vi "Set Cell_row_string.vi"(7 "Value":string, 8 "error in (no error)":errorcluster, 9 "Column":i32, 11 "Row":refnum<k24>) -> (0 "error out":errorcluster, 3 "Row Out":refnum<k24>)   [LabVIEW 2013]
uses:
  C:/PhaeronGit/LVNPOI/Resources/NPOI 2.1.1 dotnet2/NPOI.dll
  Resources/NPOI 2.1.1 dotnet2/NPOI.dll
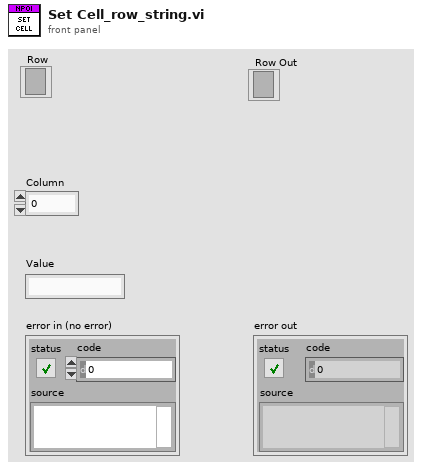
[diagram p1: front panel]
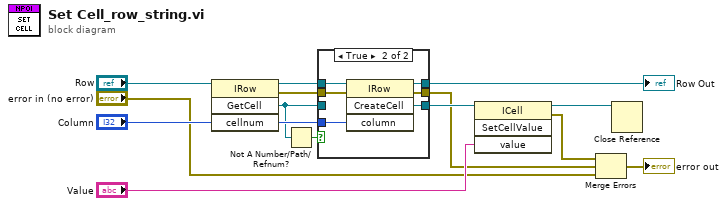
[diagram p0: block diagram]
diagram:
  n1 = invoke class="IRow" method="GetCell"(reference="Row", "cellnum"="Column") -> (reference out=w8:refnum<k24>, error out=w7:errorcluster, "GetCell"=w4:refnum<k24>)  [unwired: 2 in, 1 out]
  n2 = Not A Number/Path/Refnum?(number/path/refnum=w4) -> (NaN/Path/Refnum?=w5:bool)
  n3 = case shown="True" w5 {
    tunnel: w4 -> [w16 _]
    tunnel: [w16 w22] -> w9
    tunnel: "Column" -> [_ w21]
    tunnel: w8 -> [w15 w20]
    tunnel: [w15 w19] -> w1
    tunnel: [_ w18] -> w6
    tunnel: w7 -> [_ w17]
    frame False {
    }
    frame True {
      n4 = invoke class="IRow" method="CreateCell"(reference=w20, error in=w17, "column"=w21) -> (reference out=w19:refnum<k24>, error out=w18:errorcluster, "CreateCell"=w22:refnum<k24>)  [unwired: 1 in, 1 out]
    }
  }
  "Row Out" <- w1
  n5 = invoke class="ICell" method="SetCellValue"(reference=w9, "value"="Value") -> (reference out=w13:refnum<k24>, error out=w11:errorcluster)  [unwired: 2 in, 2 out]
  n6 = Merge Errors(w11, w6, "error in (no error)") -> (→"error out":errorcluster)
  n7 = Close Reference(reference=w13) -> ()  [unwired: 1 in, 1 out]
